vi "one button prompt message-1.vi"(8 "error in (no error)":errorcluster, 10 "Button Name (Ok)":string="Ok", 11 "Message":string) -> (0 "error out":errorcluster, 3 "OK":bool)   [LabVIEW 2022 SP3]
doc: "Displays a standard dialog box that contains an alert or a message for users.\n--------------------\n\nThis Express VI is configured as follows:\n\nMessage:"
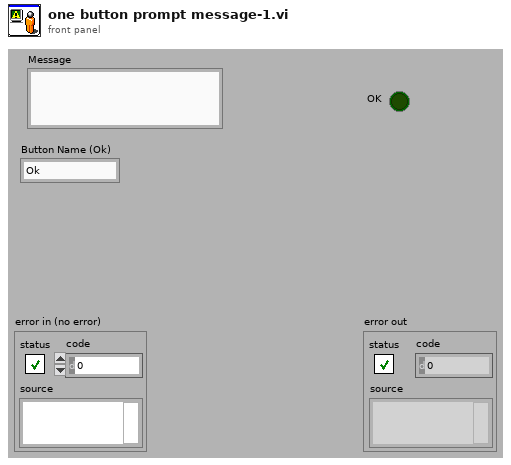
[diagram p1: front panel]
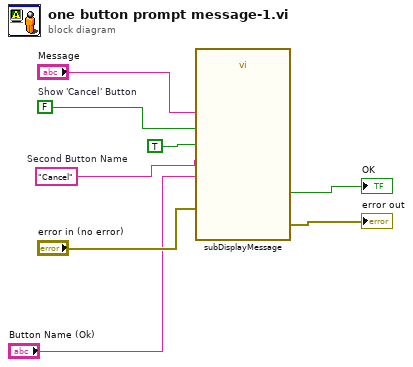
[diagram p0: block diagram]
diagram:
  w2 = "Cancel"  # Second Button Name
  w1 = FALSE  # Show 'Cancel' Button
  n1 = call <vilib>:"subDisplayMessage.vi"("Second Button Name"=w2, "Button Name"="Button Name (Ok)", "error in (no error)"="error in (no error)", "Enable Message"=TRUE, "Show 'Cancel' Button"=w1, "Message to Display"="Message") -> ("error out"=→"error out":errorcluster, "OK?"=→"OK":bool)  [unwired: 4 in]
